vi "RingValues.vi"(11 "Array":u32[](array[ring]) items=["a", "b", "c", "d", "e"]) -> (3 "Array 2":u32[](array[ring]) items=["a", "b", "c", "d", "e"])   [LabVIEW 2012]
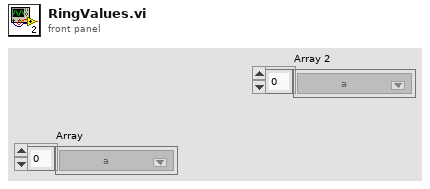
[diagram p1: front panel]
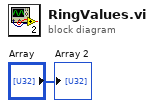
[diagram p0: block diagram]
diagram:
  "Array 2" <- "Array"
